vi "creaClasesDePruebas.vi"(8 "error in (no error)":errorcluster, 10 "NombrePruebas":string[](array[string]), 11 "Equipo in":refnum<class "Equipo.lvclass">) -> (0 "error out":errorcluster, 2 "listaDePruebas":refnum<class "Prueba.lvclass">[](array[class]), 3 "Equipo out":refnum<class "Equipo.lvclass">)   [LabVIEW 2019, in "Equipo.lvclass"]
uses:
  Equipo.lvclass
  Pruebas/Prueba/Prueba.lvclass
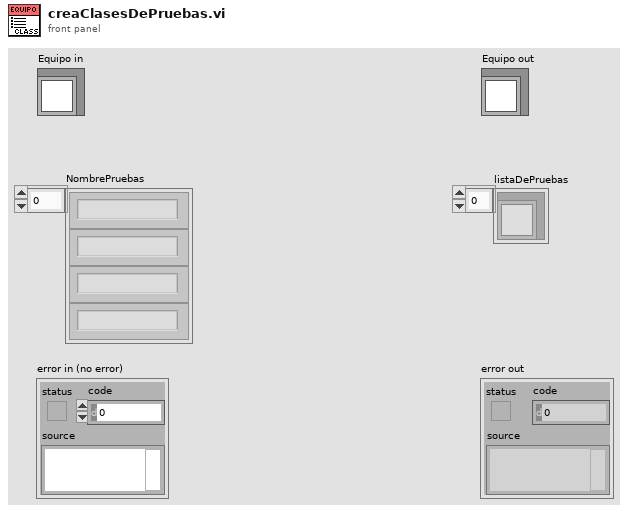
[diagram p1: front panel]
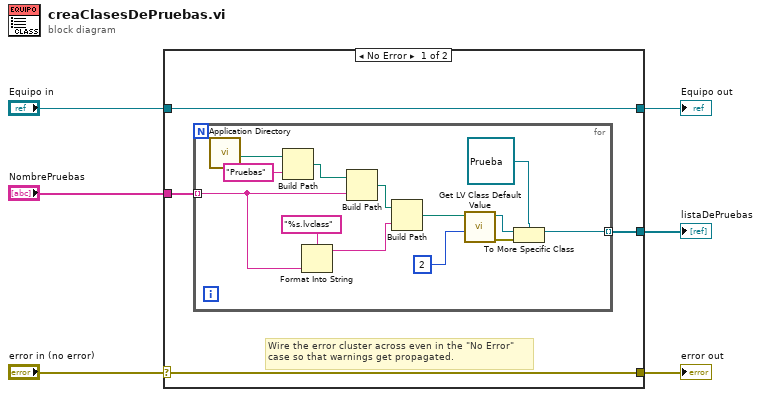
[diagram p0: block diagram]
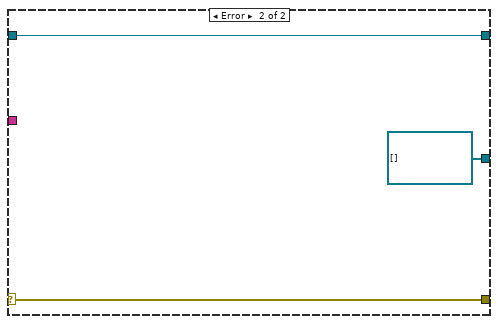
[diagram p2: hidden frame]
diagram:
  n1 = case shown="No Error" "error in (no error)" {
    selector: "error in (no error)" -> [w9 w26]
    tunnel: [w9 w26] -> w5
    tunnel: [w10 w25] -> w3
    tunnel: "Equipo in" -> [w10 w25]
    tunnel: "NombrePruebas" -> [w8 _]
    tunnel: [w7 refnum<class "Prueba.lvclass">[] []] -> w1
    frame No Error {
      # "Wire the error cluster across even in the \"No Error\"\ncase so that warnings get propagated."
      n2 = for {
        tunnel: w8 -> [w12] mode=indexing
        tunnel: [w11] -> w7 mode=indexing
        n3 = call <vilib>:"Application Directory.vi"() -> ("Application Directory"=w23:path)
        n4 = Build Path(base path=w23, name or relative path="Pruebas") -> (appended path=w21:path)
        n5 = Format Into String(format string="%s.lvclass", w12) -> (resulting string=w18:string)  [unwired: 2 in, 1 out]
        n6 = Build Path(base path=w21, name or relative path=w12) -> (appended path=w20:path)
        n7 = Build Path(base path=w20, name or relative path=w18) -> (appended path=w16:path)
        n8 = call <vilib>:"Get LV Class Default Value.vi"("options"=u32 2, "class path"=w16) -> ("error out"=w15:errorcluster, "object"=w14:refnum<class>)  [unwired: 8 in]
        n9 = To More Specific Class(target class=refnum<class "Prueba.lvclass"> refnum ("Prueba.lvclass"), reference=w14, error in=w15) -> (specific class reference=w11:refnum<class "Prueba.lvclass">)  [unwired: 1 out]
      }
    }
    frame Error {
    }
  }
  "error out" <- w5
  "Equipo out" <- w3
  "listaDePruebas" <- w1
